vi "Criar novo arquivo de configuração.vi"(2 "Path":path, 3 "Enum":T1(ring)) -> (0 "error out":errorcluster, 1 "file path":path)   [LabVIEW 2020]
uses:
  <vilib>/Utility/file.llb/Write Delimited Spreadsheet (string).vi
  <vilib>/Utility/config.llb/Write Key (String).vi
  <vilib>/Utility/config.llb/NI_LVConfig.lvlib
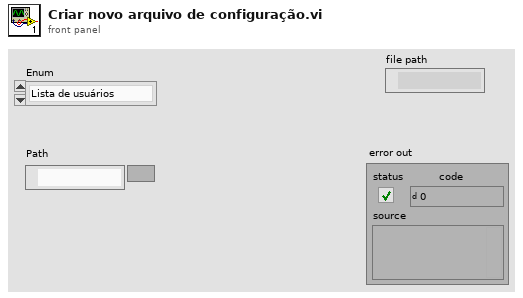
[diagram p1: front panel]
types:
  T1 = enum16{"Lista de usuários", "Configurações de máquina"}
  T2 = typedef "NI_LVConfig.lvlib/Config Data RefNum.ctl" = refnum<k1>
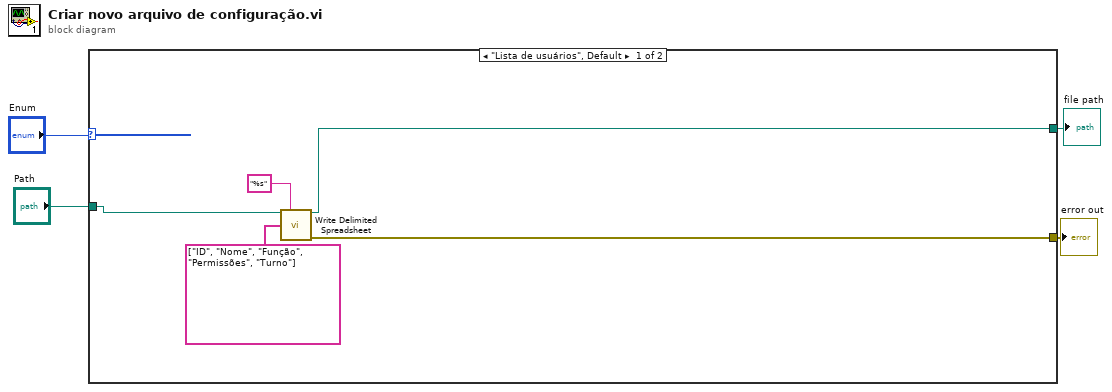
[diagram p0: block diagram]
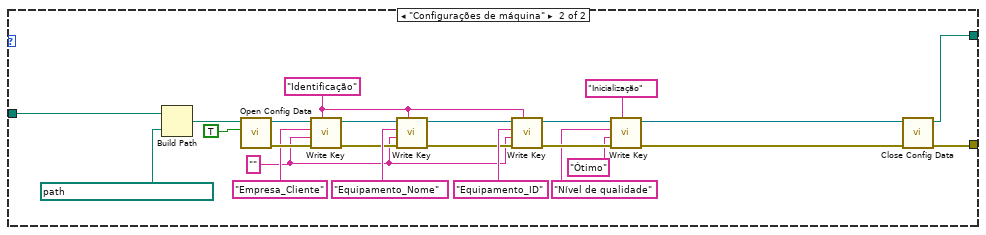
[diagram p2: hidden frame]
diagram:
  n1 = case shown="\"Lista de usuários\", Default" "Enum" {
    tunnel: "Path" -> [w5 w33]
    tunnel: [w7 w19] -> w2
    tunnel: [w6 w18] -> w1
    frame "Lista de usuários", Default {
      n2 = call-poly <vilib>:"Write Delimited Spreadsheet.vi"("file path (dialog if empty)"=w5, "format (%s)"="%s" ("format (%.3f)"), "1D data"=string[] ["ID", "Nome", "Função", "Permissões", "Turno"]) -> ("new file path (Not A Path if cancelled)"=w6:path, "error out"=w7:errorcluster)  [unwired: 11 in]
    }
    frame "Configurações de máquina" {
      w14 = ""
      w20 = "Identificação" ("section")
      n3 = Build Path(base path=w33, name or relative path=path "Configurações de máquina.ini") -> (appended path=w31:path)
      n4 = call <vilib>:"Open Config Data.vi"("create file if necessary (T)"=TRUE, "configuration file path"=w31) -> ("error out"=w28:errorcluster, "refnum"=w29:T2)  [unwired: 7 in, 1 out]
      n5 = call-poly <vilib>:"Write Key.vi"("section"=w20, "error in (no error)"=w28, "value"=w14, "key"="Empresa_Cliente", "refnum"=w29) -> ("error out"=w24:errorcluster, "refnum out"=w25:T2)  [unwired: 4 in, 1 out]
      n6 = call-poly <vilib>:"Write Key.vi"("section"=w20, "error in (no error)"=w24, "value"=w14, "key"="Equipamento_Nome", "refnum"=w25) -> ("error out"=w21:errorcluster, "refnum out"=w22:T2)  [unwired: 4 in, 1 out]
      n7 = call-poly <vilib>:"Write Key.vi"("section"=w20, "error in (no error)"=w21, "value"=w14, "key"="Equipamento_ID", "refnum"=w22) -> ("error out"=w16:errorcluster, "refnum out"=w17:T2)  [unwired: 4 in, 1 out]
      n8 = call-poly <vilib>:"Write Key.vi"("section"="Inicialização", "error in (no error)"=w16, "value"="Ótimo", "key"="Nível de qualidade", "refnum"=w17) -> ("error out"=w10:errorcluster, "refnum out"=w11:T2)  [unwired: 4 in, 1 out]
      n9 = call <vilib>:"Close Config Data.vi"("error in (no error)"=w10, "refnum"=w11) -> ("error out"=w19:errorcluster, "file path"=w18:path)  [unwired: 8 in]
    }
  }
  "error out" <- w2
  "file path" <- w1
